vi "CNT Scan Device.vi"(11 "NeedInit":u8) -> (3 "function return":i32)   [LabVIEW 2010, in "ControlCNT.lvlib"]
doc: "int WINAPI CNT_ScanDevice(unsigned char NeedInit);"
uses:
  ControlCNT.lvlib
  ControlCNT/Ginkgo_Driver.dll
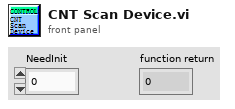
[diagram p1: front panel]
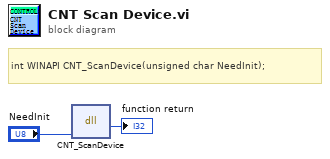
[diagram p0: block diagram]
diagram:
  # "int WINAPI CNT_ScanDevice(unsigned char NeedInit);"
  n1 = dll-call lib="E:/Project/vt_ginkgo/truck/Ginkgo Driver/vs2010/Ginkgo_USB-I2C&SPI&CAN_API_v2.0.3.3/lib/labview_32bit/ControlCNT/Ginkgo_Driver.*" fn="CNT_ScanDevice"("NeedInit"="NeedInit") -> (→"function return":i32)  [unwired: 4 in, 2 out]
